vi "获取EXCEL文档中  SHEET 名字的列表 开发环境 LABVIEW 2014版本.vi"() -> ()   [LabVIEW 2014]
panel:
  out "SHEET 的名字字符串数组":string[](array[string])
  in  "Excel._Worksheet":refnum<k7>
  in  "是否显示创建的文档":bool
  in  "error in (no error)":errorcluster
  in  "Excel._Application":refnum<k7>
  # "输入指定EXCEL文档路径  输出 该文档内部sheet 名字的字符串数组"
  # "进一步讨论：QQ470885756\n或者发邮件：wenluderen@gmail.com"
  # "工控机和上位软件讨论：20423623  主题：讨论上位系统：WINCC LABVIEW  INTOUCH MATLAB VB VC \n\n电气制图软件交流促进：182667049  主题：EPLAN  CAD PCSCHEMATIC 等\n\n电子学习共同促进群：234742235   主题：学习探讨单片机 电子线路等电子技术\n\n自动化行业非标PLC编程：170665069     主题：坦诚沟通 共同进步\n\n运动控制机器人视觉 : 254438239主题：运动控制卡：英国翠欧，美国PMAC，英国BALDOR  机器人：ABB 爱普生 三菱 雅马哈 CCD"
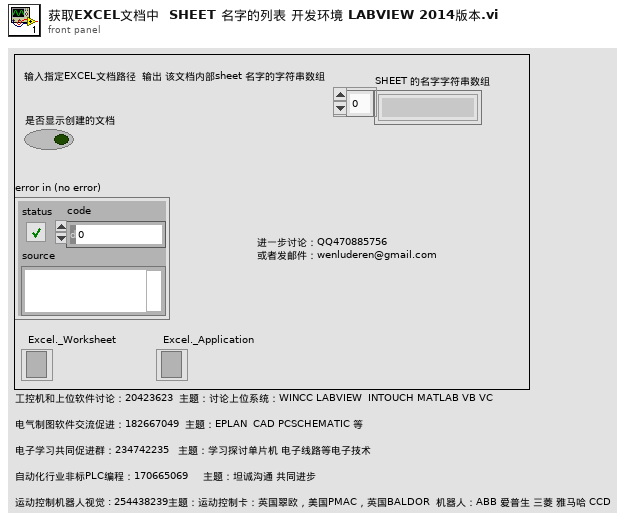
[diagram p1: front panel]
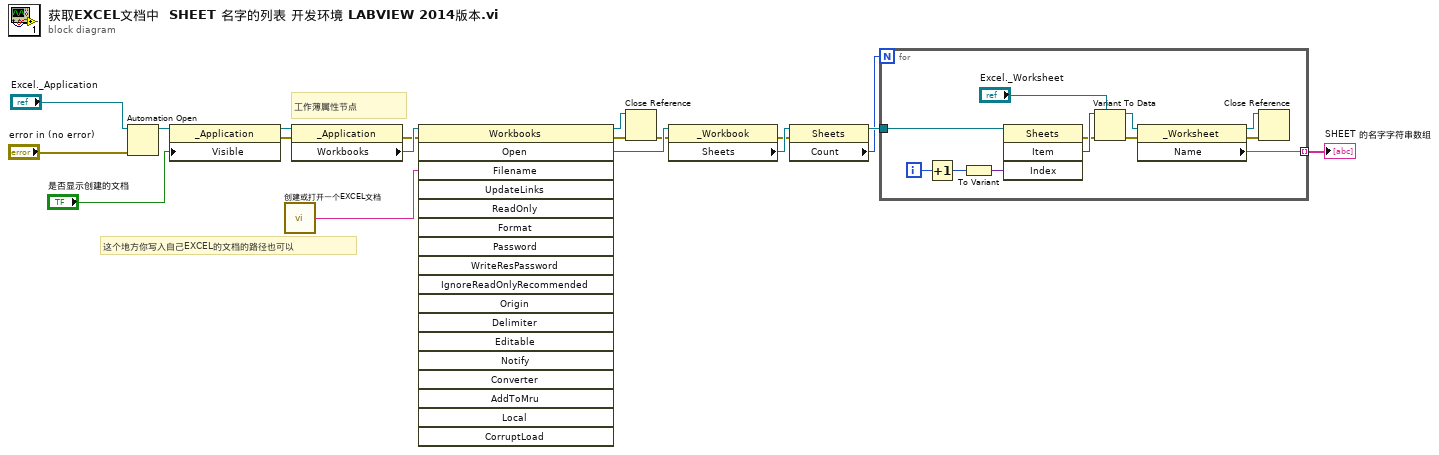
[diagram p0: block diagram]
diagram:
  # "这个地方你写入自己EXCEL的文档的路径也可以"
  # "工作薄属性节点"
  n1 = Automation Open(error in (no error)="error in (no error)", Automation Refnum="Excel._Application") -> (Automation Refnum=w16:refnum<k7>)  [unwired: 2 in, 1 out]
  n2 = property class="_Application"(reference=w16, "Visible"="是否显示创建的文档") -> (reference out=w14:refnum<k7>, error out=w13:errorcluster)  [unwired: 1 in]
  n3 = call "创建或打开一个EXCEL文档.vi"() -> ("目标文档全路径"=w10:string)  [unwired: 1 in]
  n4 = property class="_Application"(reference=w14, error in=w13) -> (error out=w11:errorcluster, "Workbooks"=w12:refnum<k7>)  [unwired: 1 out]
  n5 = invoke class="Workbooks" method="Open"(reference=w12, error in=w11, "Filename"=w10) -> (reference out=w9:refnum<k7>, error out=w8:errorcluster, "Open"=w7:refnum<k7>)  [unwired: 15 in, 15 out]
  n6 = Close Reference(reference=w9, error in (no error)=w8) -> (error out=w6:errorcluster)
  n7 = property class="_Workbook"(reference=w7, error in=w6) -> (error out=w4:errorcluster, "Sheets"=w5:refnum<k7>)  [unwired: 1 out]
  n8 = property class="Sheets"(reference=w5, error in=w4) -> (reference out=w3:refnum<k7>, "Count"=w2:i32)  [unwired: 1 out]
  n9 = for {
    N: w2 -> [_]
    tunnel: w3 -> [w30]
    tunnel: [w21] -> w1 mode=indexing
    i -> [w29]
    n10 = Increment(x=w29) -> (x+1=w27:i32)
    n11 = To Variant(anything=w27) -> (Variant=w28:variant)
    n12 = invoke class="Sheets" method="Item"(reference=w30, "Index"=w28) -> (error out=w25:errorcluster, "Item"=w26:variant)  [unwired: 2 in, 2 out]
    n13 = Variant To Data(error in=w25, type="Excel._Worksheet", Variant=w26) -> (data=w23:refnum<k7>, error out=w22:errorcluster)
    n14 = property class="_Worksheet"(reference=w23, error in=w22) -> (reference out=w20:refnum<k7>, error out=w19:errorcluster, "Name"=w21:string)
    n15 = Close Reference(reference=w20, error in (no error)=w19) -> ()  [unwired: 1 out]
  }
  "SHEET 的名字字符串数组" <- w1
